vi "CreateGroup.vi"(7 "LabVIEW Web Service Request":refnum<class "Web Request.lvclass">, 10 "accessMode":bool, 11 "groupName":string) -> ()   [LabVIEW 2013]
doc: "CreateReadGroup is used to group several tags together that all have read permissions. This allows for fast reads of all of the tags in a group. This functions similarly to the concept of a bus."
uses:
  <vilib>/wsapi/Web Request.lvclass
  <vilib>/NI/TagWebClient/API/tagweb client API.lvlib
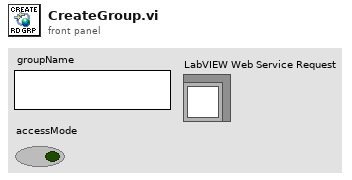
[diagram p1: front panel]
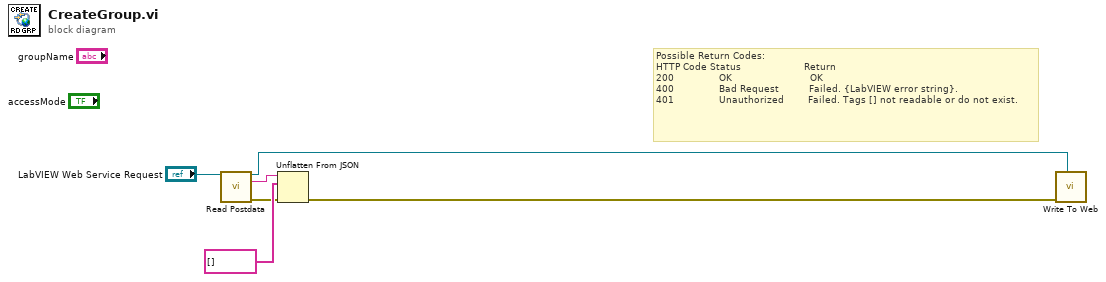
[diagram p0: block diagram]
diagram:
  # "Possible Return Codes:\nHTTP Code\tStatus\t                    Return\n200\t              OK                          OK\n400\t              Bad Request\t         Failed. {LabVIEW error string}.\n401\t              Unauthorized\t       Failed. Tags [] not readable or do not exist."
  n1 = call <vilib>:"Read Postdata.vi"("LabVIEW Web Service Request"="LabVIEW Web Service Request") -> ("LabVIEW Web Service Request out"=w5:refnum<class "Web Request.lvclass">, "postdata"=w3:string, "error out"=w2:errorcluster)  [unwired: 12 in]
  n2 = Unflatten From JSON(JSON string=w3, type and defaults=string[] [], error in (no error)=w2) -> (error out=w1:errorcluster)  [unwired: 4 in, 1 out]
  n3 = call <vilib>:"Write To Web.vi"("Web Request in"=w5, "error in"=w1) -> ()  [unwired: 10 in]
